vi "Clear.vi"(8 "error in (no error)":errorcluster, 11 "Test Runner In":refnum<class "Test Runner.lvclass">) -> (0 "error out":errorcluster, 3 "Test Runner Out":refnum<class "Test Runner.lvclass">)   [LabVIEW 2020, in "Test Runner.lvclass"]
uses:
  Test Runner.lvclass
  Application Framework/Process Classes/Process/Process.lvclass
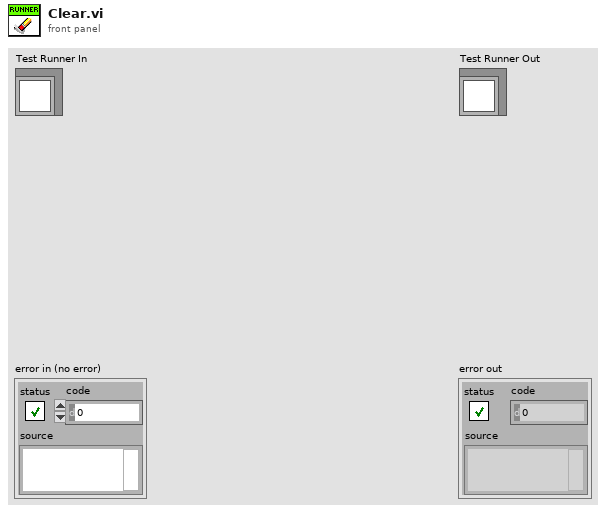
[diagram p1: front panel]
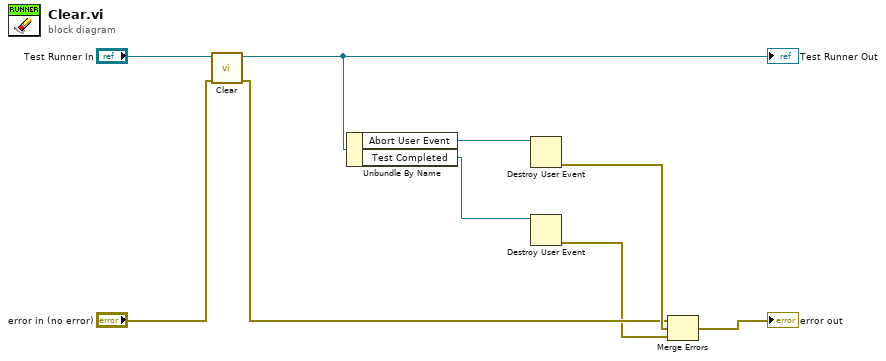
[diagram p0: block diagram]
diagram:
  n1 = call-parent "Clear.vi"("error in (no error)"="error in (no error)", "Process In"="Test Runner In") -> ("error out"=w3:errorcluster, "Process Out"=w5:refnum<class "Test Runner.lvclass">)  [unwired: 8 in]
  "Test Runner Out" <- w5
  n2 = Unbundle By Name(w5) -> ("Abort User Event"=w7:refnum<user-event>, "Test Completed"=w2:refnum<user-event>)
  n3 = Destroy User Event(user event=w7) -> (error out=w6:errorcluster)  [unwired: 1 in]
  n4 = Destroy User Event(user event=w2) -> (error out=w1:errorcluster)  [unwired: 1 in]
  n5 = Merge Errors(w3, w6, w1) -> (→"error out":errorcluster)
